vi "start.vi"(8 "error in (no error)":errorcluster, 9 "spect_depth":u16, 10 "time":sgl, 11 "identifier":string) -> (0 "error out":errorcluster, 3 "function return":u32)   [LabVIEW 2015, in "XGL_DPP.lvlib"]
doc: "EXTERN DECLSPEC uint32_t CALL_CONV start(const char * identifier, const float time, const uint16_t spect_depth);\n\n\nEXTERN DECLSPEC uint32_t CALL_CONV start(const char * identifier, const uint32_t time, const uint16_t spect_depth);\n\nEXTERN DECLSPEC uint32_t CALL_CONV start(const char * identifier, float time, const uint16_t spect_depth);"
uses:
  XGL_DPP.lvlib
  XGL_DPP.dll
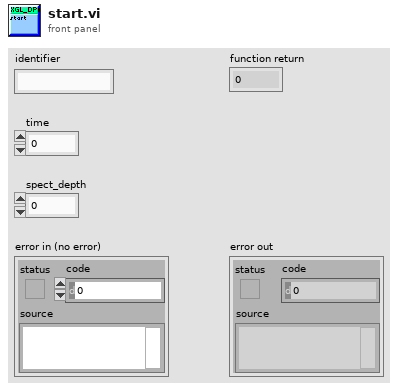
[diagram p1: front panel]
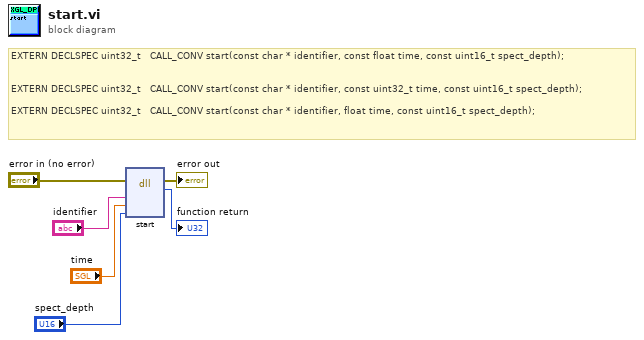
[diagram p0: block diagram]
diagram:
  # "EXTERN DECLSPEC uint32_t   CALL_CONV start(const char * identifier, const float time, const uint16_t spect_depth);\n\n\nEXTERN DECLSPEC uint32_t   CALL_CONV start(const char * identifier, const uint32_t time, const uint16_t spect_depth);\n\nEXTERN DECLSPEC uint32_t   CALL_CONV start(const char * identifier, float time, const uint16_t spect_depth);"
  n1 = dll-call lib="D:/Users/XRF/Desktop/Scanning Software_Demokritos_2015_v7/libs/Vis_2/XGL_DPP.*" fn="start"(error in="error in (no error)", "identifier"="identifier", "time"="time", "spect_depth"="spect_depth") -> (error out=→"error out":errorcluster, →"function return":u32)  [unwired: 5 in, 1 out]
